vi "SetOrigin.vi"(8 "error in (no error)":errorcluster, 11 "VI in":refnum<vi>) -> (0 "error out":errorcluster)   [LabVIEW 2018]
uses:
  <vilib>/Utility/miscctls.llb/LVPointTypeDef.ctl
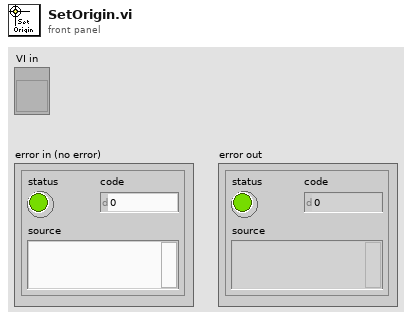
[diagram p1: front panel]
types:
  T1 = typedef "LVPointTypeDef.ctl" = cluster{"Horizontal":i16, "Vertical":i16}
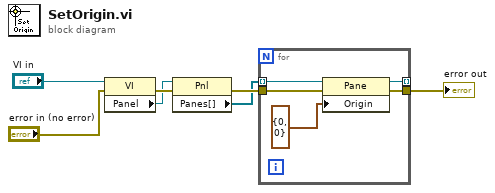
[diagram p0: block diagram]
diagram:
  n1 = property class="VI"(reference="VI in", error in="error in (no error)") -> (error out=w5:errorcluster, "Panel"=w4:refnum<vi>)  [unwired: 1 out]
  n2 = property class="Pnl"(reference=w4, error in=w5) -> (error out=w7:errorcluster, "Panes[]"=w6:refnum<vi>[])  [unwired: 1 out]
  n3 = for {
    tunnel: w6 -> [w12] mode=indexing
    tunnel: w7 -> [w11]
    tunnel: [w9] -> w1
    tunnel: [w8] -> _ mode=indexing
    n4 = property class="Pane"(reference=w12, error in=w11, "Origin"=T1 {"Horizontal"=0, "Vertical"=0}) -> (reference out=w8:refnum<vi>, error out=w9:errorcluster)
  }
  "error out" <- w1
